vi "AS2.vi"() -> ()   [LabVIEW 2025]
uses:
  State.ctl
  Main clusterer.ctl
  Button enable-disabel.ctl
  <vilib>/gmath/NI_Gmath.lvlib
panel:
  in  "FFT":bool
  in  "(X/Y)-Axis":bool
  in  "Z-Axis":bool
  out "Tab":enum32{"Z-Axis", "(X/Y)-Axis", "FFT"}(tab)
  out "Waveform Chart":cluster{"Numeric":dbl, "Scalar":dbl}(graph)
  out "Waveform Chart 2":cluster{"Numeric":dbl, "Scalar":dbl}(graph)
  in  "Interpolation method":T1(ring)=enum."linear"
  in  "Calibration":bool
  in  "Finish measurement":bool
  in  "Save Button":bool
  in  "Stop Button":bool
  in  "Start":bool
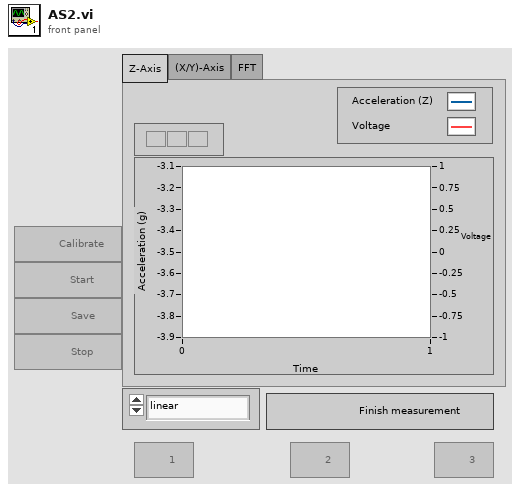
[diagram p1: front panel]
types:
  T1 = enum16{"nearest", "linear", "spline", "cubic Hermite", "Lagrange"}
  T2 = typedef "Main clusterer.ctl" = cluster{"Acceleration (X/Y) [g] | Voltage [V]":dbl[][], "Measured (X/Y) acceleration":dbl[], "Acceleration (Z) [g] | Voltage [V] 2":dbl[][], "Measured (Z) acceleration":dbl[]}
  T3 = typedef "State.ctl" = enum16{"Initialize", "Calibrate", "Wait for Event", "Start", "Stop", "Save"}
  T4 = typedef "Button enable-disabel.ctl" = enum8{"Enabled", "Disabled", "Disabled and Grayed Out"}
  T5 = cluster{"Distance [cm]| Voltage [V]":dbl[][], "Measured (X/Y) acceleration":dbl[], "Distance [cm]| Voltage [V]":dbl[][], "Measured (Z) acceleration":dbl[]}
  T6 = cluster{"Acceleration (X/Y) [g] | Voltage [V]":dbl[][], dbl[], "Acceleration (Z) [g] | Voltage [V] 2":dbl[][], dbl[]}
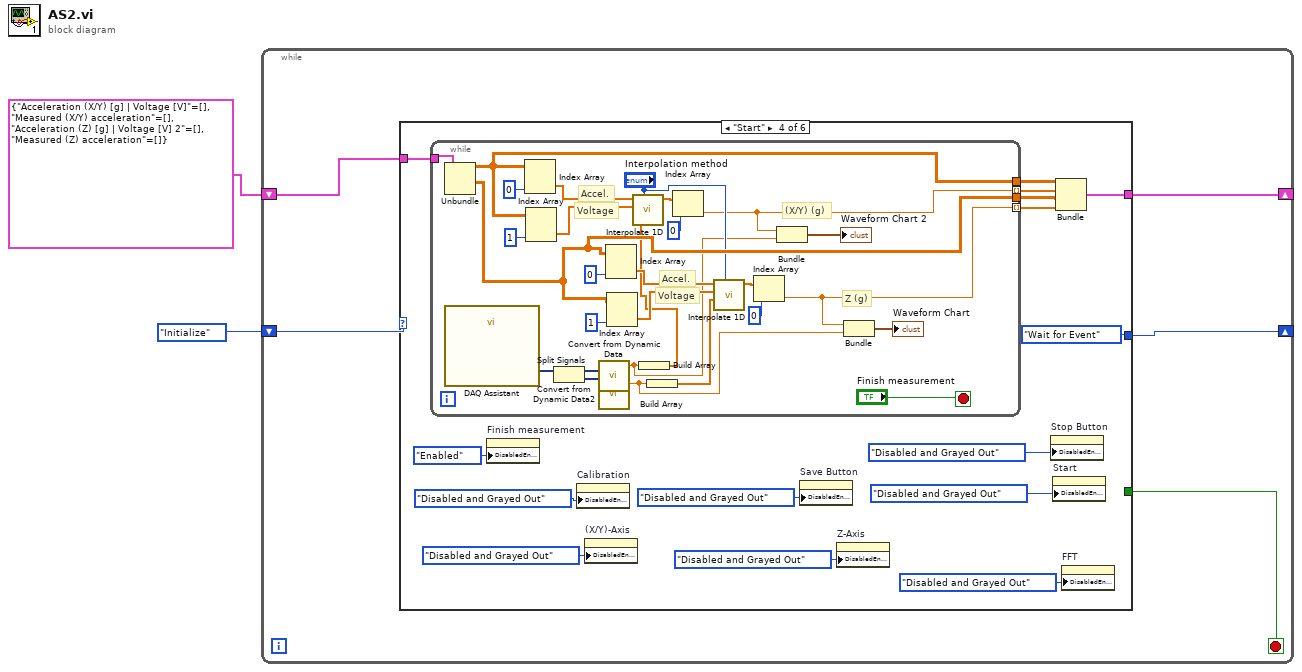
[diagram p0: block diagram]
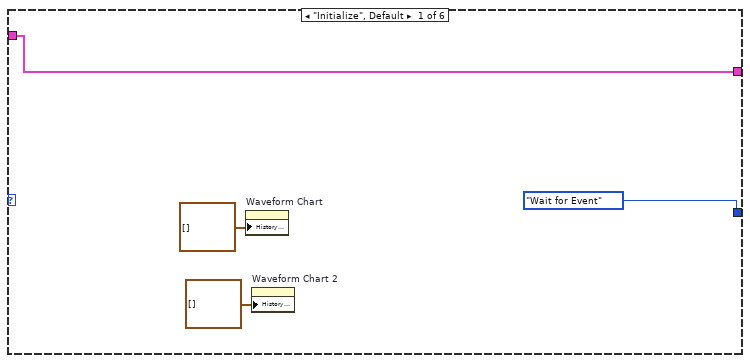
[diagram p2: hidden frame]
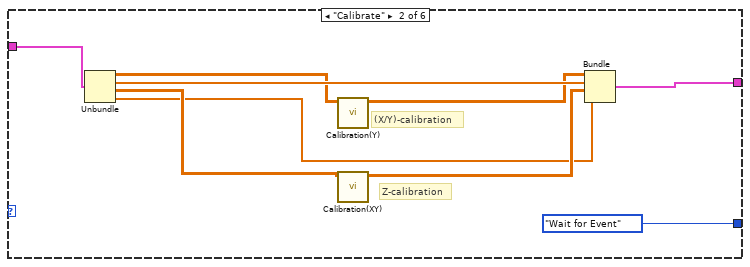
[diagram p3: hidden frame]
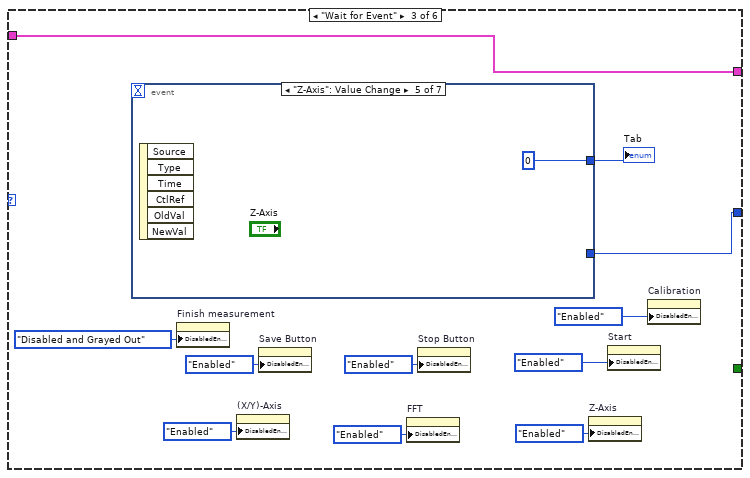
[diagram p4: hidden frame]
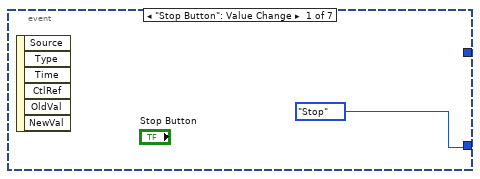
[diagram p5: hidden frame]
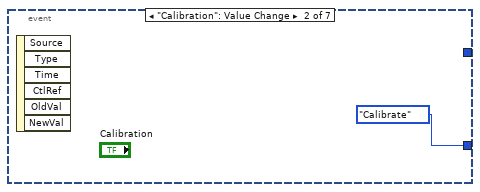
[diagram p6: hidden frame]
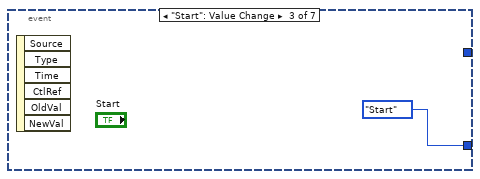
[diagram p7: hidden frame]
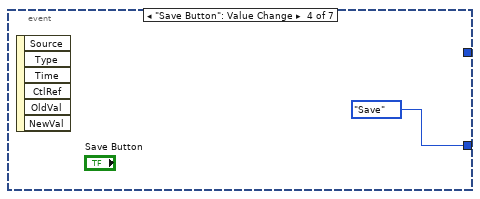
[diagram p8: hidden frame]
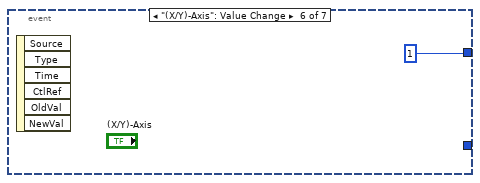
[diagram p9: hidden frame]
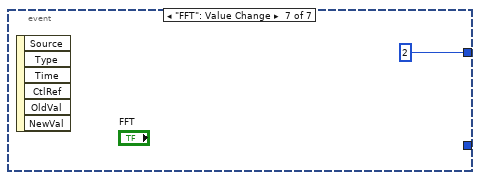
[diagram p10: hidden frame]
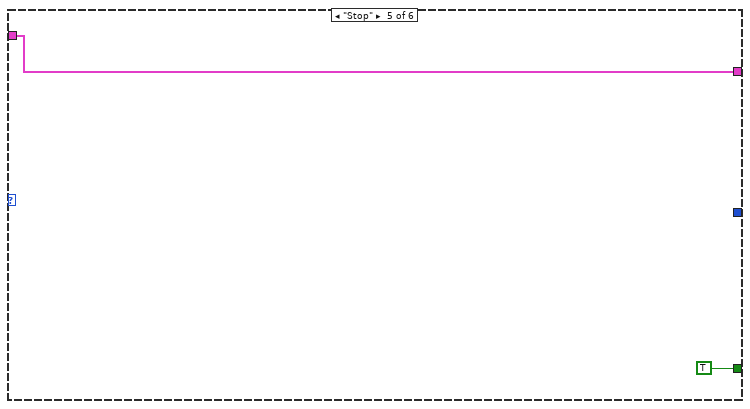
[diagram p11: hidden frame]
diagram:
  n1 = while {
    shift-right: [w4] -> _
    shift-left: State."Initialize" ("State") -> [w7]
    shift-right: [w5] -> _
    shift-left: T2 {"Acceleration (X/Y) [g] | Voltage [V]"=[], "Measured (X/Y) acceleration"=[], "Acceleration (Z) [g] | Voltage [V] 2"=[], "Measured (Z) acceleration"=[]} ("Main cluster") -> [w6]
    stop <- w3 stop-if-true
    n2 = case shown="\"Start\"" w7 {
      tunnel: w6 -> [w10 w20 w27 w47 w82 w84]
      tunnel: [w10 w18 w27 w46 w82 w84] -> w5
      tunnel: [State."Wait for Event" ("State") State."Wait for Event" ("State") w26 State."Wait for Event" ("State") _ _] -> w4
      tunnel: [_ _ _ _ TRUE _] -> w3
      frame "Initialize", Default {
        n3 = property on="Waveform Chart" class="WFChart (strict)"("History Data"=cluster{"Numeric":dbl, "Scalar":dbl}[] []) -> ()  [unwired: 2 in, 2 out]
        n4 = property on="Waveform Chart 2" class="WFChart (strict)"("History Data"=cluster{"Numeric":dbl, "Scalar":dbl}[] []) -> ()  [unwired: 2 in, 2 out]
      }
      frame "Calibrate" {
        # "Z-calibration"
        # "(X/Y)-calibration"
        n5 = Unbundle(w20) -> ("Acceleration (X/Y) [g] | Voltage [V]"=w16:dbl[][], "Measured (X/Y) acceleration"=w19:dbl[], "Acceleration (Z) [g] | Voltage [V] 2"=w17:dbl[][], "Measured (Z) acceleration"=w12:dbl[])
        n6 = call "Calibration(Y).vi"("Acceleration [g]| Voltage [V]"=w16) -> ("Distance [cm]| Voltage [V]"=w15:dbl[][])  [unwired: 8 in, 2 out]
        n7 = call "Calibration(XY).vi"("Acceleration [g]| Voltage [V]"=w17) -> ("Distance [cm]| Voltage [V]"=w13:dbl[][])  [unwired: 8 in, 2 out]
        n8 = Bundle("Distance [cm]| Voltage [V]"=w15, "Measured (X/Y) acceleration"=w19, "Distance [cm]| Voltage [V]"=w13, "Measured (Z) acceleration"=w12) -> (w18:T5)  [unwired: 1 in]
      }
      frame "Wait for Event" {
        n9 = event shown="[4] \"Z-Axis\": Value Change" {
          selector: _ -> [_ _ _ _ _ _ _]
          dyn-events: _ -> [_ _ _ _ _ _ _]
          timeout: _ -> [_ _ _ _ _ _ _]
          tunnel: [State."Stop" ("State") State."Calibrate" ("State") State."Start" ("State") State."Save" ("State") _ _ _] -> w26
          tunnel: [_ _ _ _ 0 1 2] -> w24
          event "Stop Button": Value Change {
            n10 = event-data() -> ()  [unwired: 1 in, 6 out]
          }
          event "Calibration": Value Change {
            n11 = event-data() -> ()  [unwired: 1 in, 6 out]
          }
          event "Start": Value Change {
            n12 = event-data() -> ()  [unwired: 1 in, 6 out]
          }
          event "Save Button": Value Change {
            n13 = event-data() -> ()  [unwired: 1 in, 6 out]
          }
          event "Z-Axis": Value Change {
            n14 = event-data() -> ()  [unwired: 1 in, 6 out]
          }
          event "(X/Y)-Axis": Value Change {
            n15 = event-data() -> ()  [unwired: 1 in, 6 out]
          }
          event "FFT": Value Change {
            n16 = event-data() -> ()  [unwired: 1 in, 6 out]
          }
        }
        "Tab" <- w24
        n17 = property on="Finish measurement" class="Bool"("DisabledEnum"=Button_enable-disabel."Disabled and Grayed Out" ("Disabled")) -> ()  [unwired: 2 in, 2 out]
        n18 = property on="(X/Y)-Axis" class="Bool"("DisabledEnum"=Button_enable-disabel."Enabled" ("Disabled")) -> ()  [unwired: 2 in, 2 out]
        n19 = property on="Save Button" class="Bool"("DisabledEnum"=Button_enable-disabel."Enabled" ("Disabled")) -> ()  [unwired: 2 in, 2 out]
        n20 = property on="FFT" class="Bool"("DisabledEnum"=Button_enable-disabel."Enabled" ("Disabled")) -> ()  [unwired: 2 in, 2 out]
        n21 = property on="Stop Button" class="Bool"("DisabledEnum"=Button_enable-disabel."Enabled" ("Disabled")) -> ()  [unwired: 2 in, 2 out]
        n22 = property on="Z-Axis" class="Bool"("DisabledEnum"=Button_enable-disabel."Enabled" ("Disabled")) -> ()  [unwired: 2 in, 2 out]
        n23 = property on="Start" class="Bool"("DisabledEnum"=Button_enable-disabel."Enabled" ("Disabled")) -> ()  [unwired: 2 in, 2 out]
        n24 = property on="Calibration" class="Bool"("DisabledEnum"=Button_enable-disabel."Enabled" ("Disabled")) -> ()  [unwired: 2 in, 2 out]
      }
      frame "Start" {
        n25 = while {
          tunnel: w47 -> [w80]
          tunnel: [w65] -> w45
          tunnel: [w62] -> w44 mode=indexing
          tunnel: [w64] -> w43
          tunnel: [w60] -> w42 mode=indexing
          stop <- "Finish measurement" stop-if-true
          # "(X/Y) (g)"
          # "Z (g)"
          # "Accel."
          # "Voltage"
          # "Accel."
          # "Voltage"
          n26 = Unbundle(w80) -> ("Acceleration (X/Y) [g] | Voltage [V]"=w65:dbl[][], "Acceleration (Z) [g] | Voltage [V] 2"=w64:dbl[][])  [unwired: 2 out]
          n27 = call "DAQ Assistant"() -> ("data"=w54:dynamicdata)  [unwired: 17 in, 2 out]
          n28 = Index Array(array=w65, index (col)=0 ("disabled index (col)")) -> (element=w77:dbl[])  [unwired: 1 in]
          n29 = Index Array(array=w65, index (col)=1 ("disabled index (col)")) -> (element=w76:dbl[])  [unwired: 1 in]
          n30 = Split Signals(w54) -> (w67:dynamicdata, w66:dynamicdata)  [unwired: 2 in]
          n31 = call "Convert from Dynamic Data"("Dynamic Data Type"=w67) -> ("Scalar"=w58:dbl)  [unwired: 3 in]
          n32 = call "Convert from Dynamic Data2"("Dynamic Data Type"=w66) -> ("Scalar"=w57:dbl)  [unwired: 3 in]
          n33 = Index Array(array=w64, index (col)=0 ("disabled index (col)")) -> (element=w71:dbl[])  [unwired: 1 in]
          n34 = Index Array(array=w64, index (col)=1 ("disabled index (col)")) -> (element=w70:dbl[])  [unwired: 1 in]
          n35 = Build Array(w58) -> (w61:dbl[])
          n36 = call <vilib>:"Interpolate 1D.vi"("method"="Interpolation method", "xi"=w61, "X"=w76, "Y"=w77) -> ("yi"=w75:dbl[])  [unwired: 5 in, 2 out]
          n37 = Build Array(w57) -> (w59:dbl[])
          n38 = Index Array(array=w75, index=0) -> (element=w62:dbl)
          n39 = call <vilib>:"Interpolate 1D.vi"("method"="Interpolation method", "xi"=w59, "X"=w70, "Y"=w71) -> ("yi"=w69:dbl[])  [unwired: 5 in, 2 out]
          n40 = Index Array(array=w69, index=0) -> (element=w60:dbl)
          n41 = Bundle("Numeric"=w62, "Scalar"=w58) -> (→"Waveform Chart 2":cluster{"Numeric":dbl, "Scalar":dbl})  [unwired: 1 in]
          n42 = Bundle("Numeric"=w60, "Scalar"=w57) -> (→"Waveform Chart":cluster{"Numeric":dbl, "Scalar":dbl})  [unwired: 1 in]
        }
        n43 = property on="Finish measurement" class="Bool"("DisabledEnum"=Button_enable-disabel."Enabled" ("Disabled")) -> ()  [unwired: 2 in, 2 out]
        n44 = property on="Calibration" class="Bool"("DisabledEnum"=Button_enable-disabel."Disabled and Grayed Out" ("Disabled")) -> ()  [unwired: 2 in, 2 out]
        n45 = property on="(X/Y)-Axis" class="Bool"("DisabledEnum"=Button_enable-disabel."Disabled and Grayed Out" ("Disabled")) -> ()  [unwired: 2 in, 2 out]
        n46 = property on="Save Button" class="Bool"("DisabledEnum"=Button_enable-disabel."Disabled and Grayed Out" ("Disabled")) -> ()  [unwired: 2 in, 2 out]
        n47 = property on="Z-Axis" class="Bool"("DisabledEnum"=Button_enable-disabel."Disabled and Grayed Out" ("Disabled")) -> ()  [unwired: 2 in, 2 out]
        n48 = property on="Stop Button" class="Bool"("DisabledEnum"=Button_enable-disabel."Disabled and Grayed Out" ("Disabled")) -> ()  [unwired: 2 in, 2 out]
        n49 = property on="Start" class="Bool"("DisabledEnum"=Button_enable-disabel."Disabled and Grayed Out" ("Disabled")) -> ()  [unwired: 2 in, 2 out]
        n50 = Bundle("Acceleration (X/Y) [g] | Voltage [V]"=w45, w44, "Acceleration (Z) [g] | Voltage [V] 2"=w43, w42) -> (w46:T6)  [unwired: 1 in]
        n51 = property on="FFT" class="Bool"("DisabledEnum"=Button_enable-disabel."Disabled and Grayed Out" ("Disabled")) -> ()  [unwired: 2 in, 2 out]
      }
      frame "Stop" {
      }
      frame "Save" {
      }
    }
  }
